vi "File_SetValues.vi"(8 "error in (no error)":errorcluster, 10 "Data In":dbl[](array[numeric]), 11 "File in":refnum<class "File.lvclass">) -> (0 "error out":errorcluster, 3 "File out":refnum<class "File.lvclass">)   [LabVIEW 2023, in "File.lvclass"]
doc: "Sets the values of the single value channels given their order and an ordered set of doubles."
uses:
  File.lvclass
  File.lvclass/File.ctl
  Group/Group.lvclass
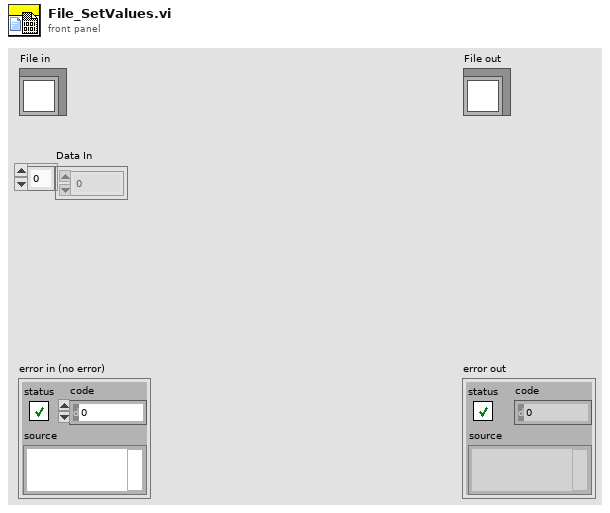
[diagram p1: front panel]
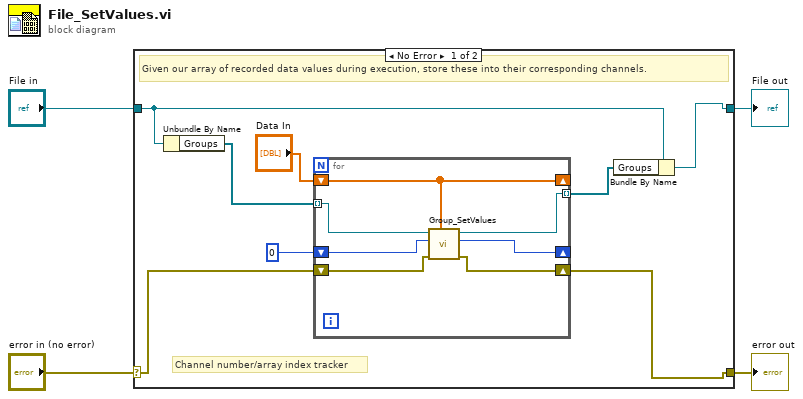
[diagram p0: block diagram]
diagram:
  n1 = case shown="No Error" "error in (no error)" {
    selector: "error in (no error)" -> [w11 w21]
    tunnel: [w8 w21] -> w3
    tunnel: [w10 w20] -> w1
    tunnel: "File in" -> [w9 w20]
    frame No Error {
      # "Channel number/array index tracker"
      # "Given our array of recorded data values during execution, store these into their corresponding channels."
      n2 = Unbundle By Name(w9) -> ("Groups"=w12:refnum<class "Group.lvclass">[])
      n3 = for {
        tunnel: w12 -> [w19] mode=indexing
        shift-right: [w17] -> w8
        shift-left: w11 -> [w16]
        tunnel: [w18] -> w7 mode=indexing
        shift-right: [w13] -> _
        shift-left: 0 -> [w14]
        shift-right: [w15] -> _
        shift-left: "Data In" -> [w15]
        n4 = call-dynamic "Group_SetValues.vi"("Data In"=w15, "error in (no error)"=w16, "Channel Count In"=w14, "Group in"=w19) -> ("error out"=w17:errorcluster, "Channel Count Out"=w13:u32, "Group out"=w18:refnum<class "Group.lvclass">)  [unwired: 5 in]
      }
      n5 = Bundle By Name(cluster=w9, "Groups"=w7) -> (w10:refnum<class "File.lvclass">)
    }
    frame Error {
    }
  }
  "error out" <- w3
  "File out" <- w1
